vi "geometry.vi"(8 "Error In":errorcluster, 11 "QWindow In":refnum<class "QWindow.lvclass">) -> (0 "Error Out":errorcluster, 2 "Value":T1, 3 "QWindow Out":refnum<class "QWindow.lvclass">)   [LabVIEW 2014, in "QWindow.lvclass"]
doc: "LabVIEW-specific documentation is not yet available. See <b>http://doc.qt.io/qt-5/QWindow.html#geometry</b>"
uses:
  QWindow.lvclass
  LQ Core/QRect.ctl
  LQ Core/LQIdentity/LQIdentity.lvclass/LQIdentity.ctl
  LQ Core/LQ Core.lvlib
  LQ Core/LQIdentity/LQIdentity.lvclass
panel:
  # "Copyright (c) 2016 Sze Howe Koh\n\nThis Source Code Form is subject to the terms of the Mozilla Public\nLicense, v. 2.0. If a copy of the MPL was not distributed with this\nfile, You can obtain one at http://mozilla.org/MPL/2.0/."
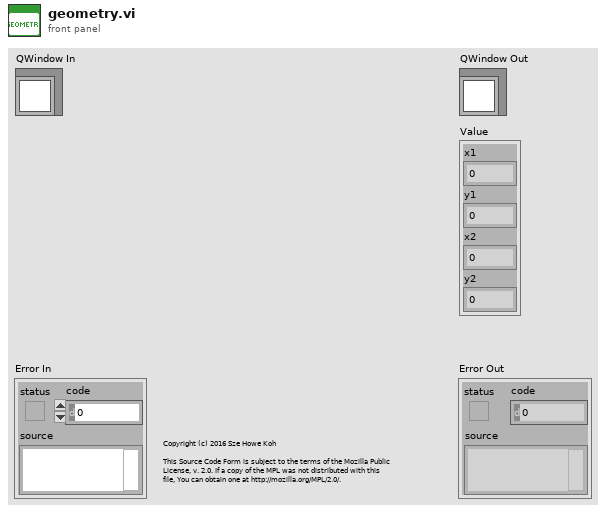
[diagram p1: front panel]
types:
  T1 = typedef "QRect.ctl" = cluster{"x1":i32, "y1":i32, "x2":i32, "y2":i32}
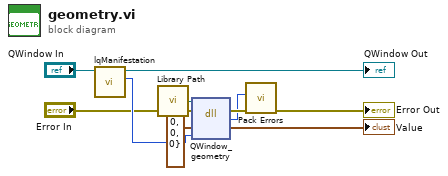
[diagram p0: block diagram]
diagram:
  n1 = call "lqManifestation.vi"("LQIdentity in"="QWindow In") -> ("Manifestation"=w5:u64, "LQIdentity out"=→"QWindow Out":refnum<class "QWindow.lvclass">)  [unwired: 9 in]
  n2 = call "Library Path.vi"() -> ("Library Path"=w6:path)
  n3 = dll-call lib="?" fn="QWindow_geometry"(path in=w6, error in="Error In", "_retVal"=T1 {"x1"=0, "y1"=0, "x2"=0, "y2"=0} ("retVal"), "_instance"=w5) -> (error out=w3:errorcluster, w1:i32, "_retVal"=→"Value":T1)  [unwired: 2 in, 1 out]
  n4 = call "Pack Errors.vi"("Error In"=w3, "Error Code"=w1) -> ("Error Out"=→"Error Out":errorcluster)  [unwired: 9 in]
